vi "re_LuaVIEW Registry Daemon.vi"   [LabVIEW 2012]
doc: "This daemon opens references to public function VIs and manages the public registry. By running in the background it prevents LabVIEW from prematurely closing those references, which happens when the top-level context in which the reference was opened terminates. This daemon is messaged via the \"Daemon Exchange\" object.\n\nThis VI is reentrant so that it can be prepared for a reentrant run which allows it to be run even though it is included into the hierarchy via a static VI reference."
uses:
  typedefs/t_LuaVIEW Registry Daemon States.ctl
  typedefs/t_LuaVIEW Daemon Exchange Methods.ctl
  typedefs/t_LuaVIEW CIN Spinlocked Actions.ctl
  typedefs/t_LuaVIEW Reference.ctl
types:
  T1 = typedef "t_LuaVIEW Daemon Exchange Methods.ctl" = enum16{"inert", "send path", "send cleanup", "get sent", "reply", "get reply", "unset launched"}
  T2 = typedef "t_LuaVIEW Registry Daemon States.ctl" = enum16{"empty queue", "handle message", "exit LabVIEW", "initialize", "cleanup tasks", "cleanup", "stop"}
  T3 = typedef "t_LuaVIEW CIN Spinlocked Actions.ctl" = enum16{"totals", "taskcount", "open", "registerpublic", "registerexport", "revokeexports", "unregnextpublic", "usepublic", "pollexport", "close", "startyieldtest", "endyieldtest", "pollprintbuffer"}
  T4 = typedef "t_LuaVIEW Reference.ctl" = refnum<k1>
  T5 = typedef "et_LuaVIEW CIN Results.ctl" = enum16{"OK", "error", "main", "call", "clonecall", "modulecall", "exportcall", "index", "yield"}
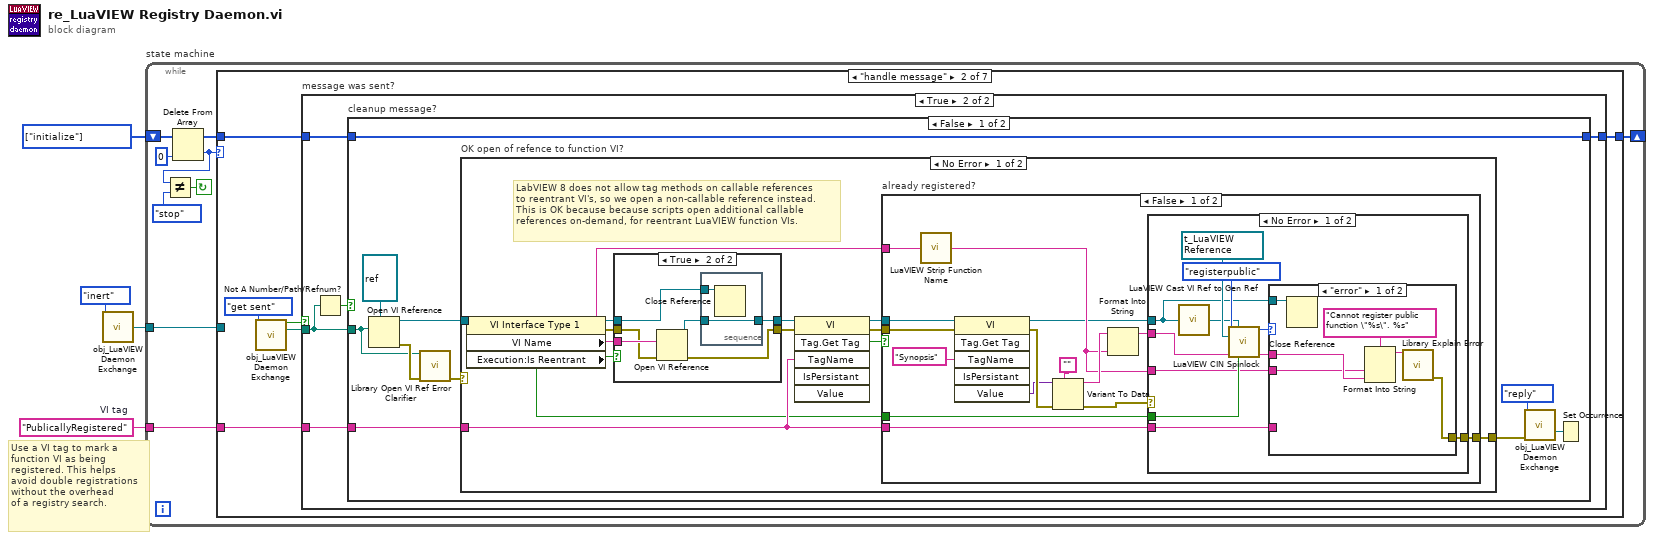
[diagram p0: block diagram]
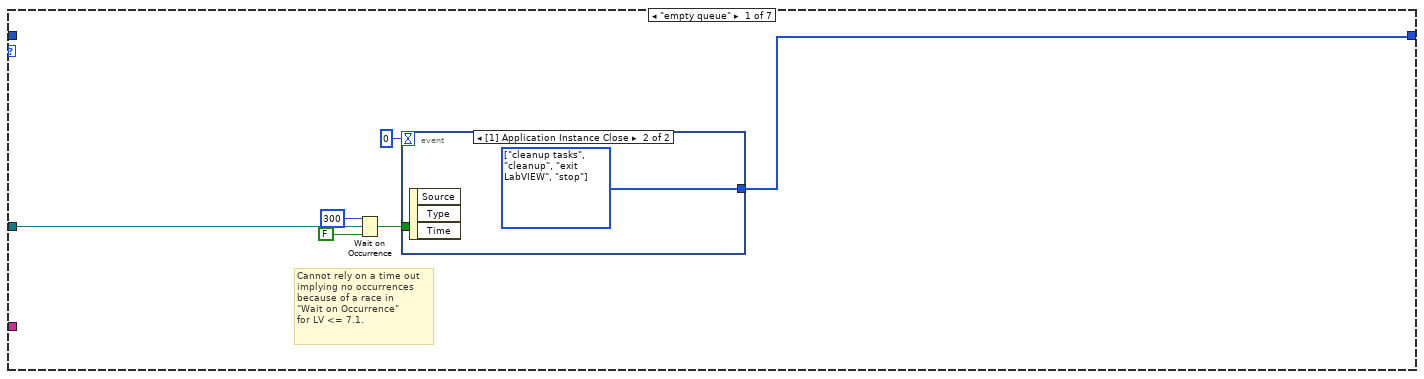
[diagram p2: hidden frame]
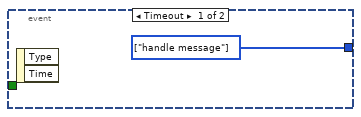
[diagram p3: hidden frame]
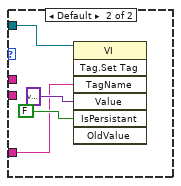
[diagram p6: hidden frame]
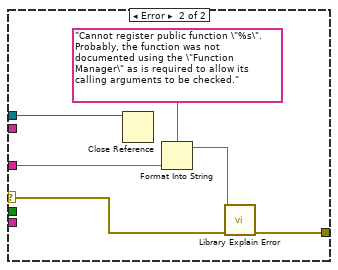
[diagram p7: hidden frame]
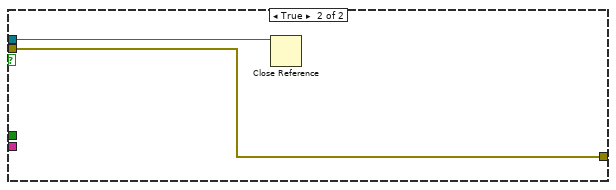
[diagram p8: hidden frame]
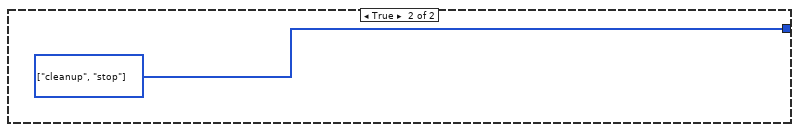
[diagram p10: hidden frame]
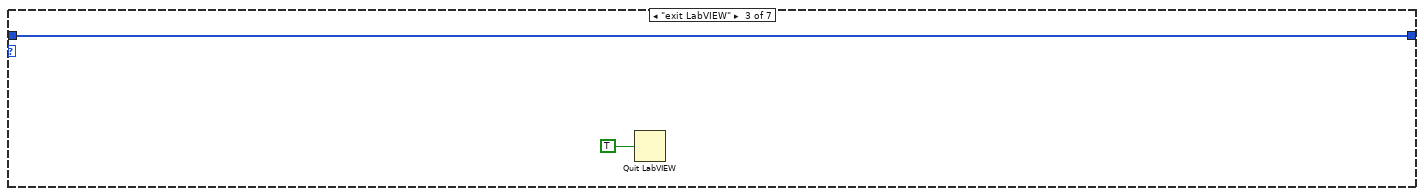
[diagram p11: hidden frame]
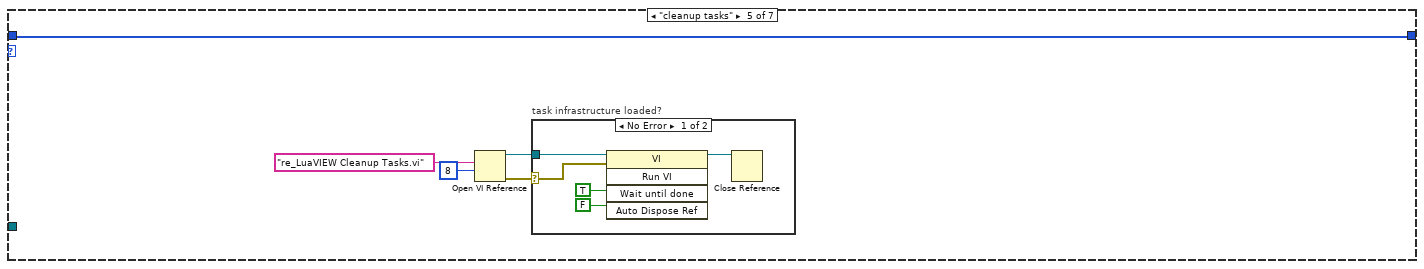
[diagram p13: hidden frame]
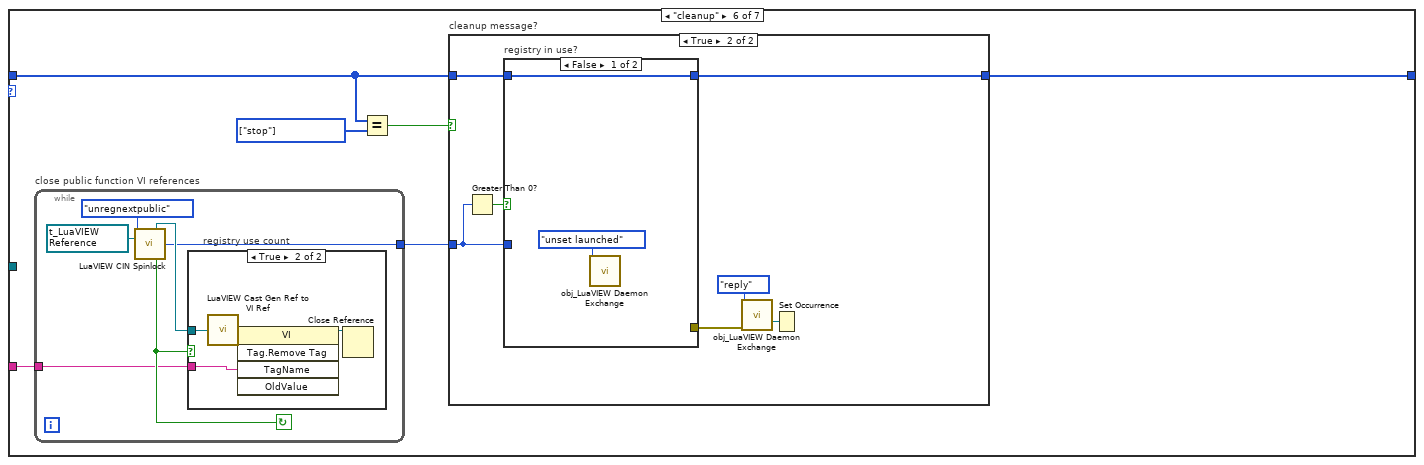
[diagram p15: hidden frame]
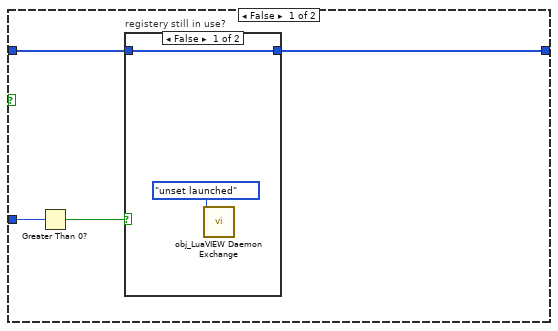
[diagram p16: hidden frame]
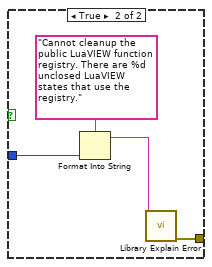
[diagram p18: hidden frame]
diagram:
  w1 = "PublicallyRegistered"  # VI tag
  w4 = T2[] [enum."initialize"] items=["empty queue", "handle message", "exit LabVIEW", "initialize", "cleanup tasks", "cleanup", "stop"] ("Array Constant")
  # "Use a VI tag to mark a\nfunction VI as being\nregistered. This helps\navoid double registrations\nwithout the overhead\nof a registry search."
  n1 = call "obj_LuaVIEW Daemon Exchange.vi"("method"=t_LuaVIEW_Daemon_Exchange_Methods."inert") -> ("send occurrence"=w2:refnum<k4>)  [unwired: 10 in, 4 out]
  n2 = while "state machine" {
    shift-left: w4 -> [w10]
    shift-right: [w13] -> _
    tunnel: w2 -> [w6]
    tunnel: w1 -> [w5]
    stop <- w12 continue-if-true
    n3 = Delete From Array(array=w10, index=0) -> (deleted portion=w8:T2, array with subset deleted=w9:T2[])  [unwired: 1 in]
    n4 = Not Equal?(x=w8, y=t_LuaVIEW_Registry_Daemon_States."stop" ("states")) -> (x != y?=w12:bool)
    n5 = case "Case" shown="\"handle message\"" w8 {
      tunnel: [w16 w23 w113 w114 w119 w130 w160] -> w13
      tunnel: w9 -> [_ w24 w113 w114 w119 w128 w160]
      tunnel: w6 -> [w17 _ _ _ _ _ _]
      tunnel: w5 -> [_ w22 _ _ _ w129 _]
      frame "empty queue" {
        # "Cannot rely on a time out\nimplying no occurrences\nbecause of a race in\n\"Wait on Occurrence\"\nfor LV <= 7.1."
        n6 = Wait on Occurrence(1:FALSE ("ignore previous (T)"), 2:w17, 3:300 ("ms timeout (-1)")) -> (0:w14:bool)
        n7 = event shown="[1] Application Instance Close" {
          selector: _ -> [_ _]
          dyn-events: _ -> [_ _]
          timeout: 0 -> [_ _]
          tunnel: [w20 w21] -> w16
          tunnel: w14 -> [_ _]
          event Timeout {
            w20 = T2[] [enum."handle message"] items=["empty queue", "handle message", "exit LabVIEW", "initialize", "cleanup tasks", "cleanup", "stop"] ("Array Constant")
            n8 = event-data() -> ()  [unwired: 1 in, 2 out]
          }
          event Application Instance Close {
            w21 = T2[] [enum."cleanup tasks", enum."cleanup", enum."exit LabVIEW", enum."stop"] items=["empty queue", "handle message", "exit LabVIEW", "initialize", "cleanup tasks", "cleanup", "stop"] ("Array Constant")
            n9 = event-data() -> ()  [unwired: 1 in, 3 out]
          }
        }
      }
      frame "handle message" {
        n10 = call "obj_LuaVIEW Daemon Exchange.vi"("method"=t_LuaVIEW_Daemon_Exchange_Methods."get sent") -> ("available?"=w25:bool, "path out"=w26:path)  [unwired: 10 in, 3 out]
        n11 = case "message was sent?" shown="True" w25 {
          tunnel: w26 -> [_ w31]
          tunnel: w24 -> [w28 w33]
          tunnel: [w28 w32] -> w23
          tunnel: w22 -> [_ w29]
          frame False {
          }
          frame True {
            n12 = Not A Number/Path/Refnum?(number/path/refnum=w31) -> (NaN/Path/Refnum?=w30:bool)
            n13 = case "cleanup message?" shown="False" w30 {
              tunnel: w31 -> [w42 _]
              tunnel: w33 -> [w41 _]
              tunnel: [w41 w111] -> w32
              tunnel: w29 -> [w38 _]
              frame False {
                n14 = Open VI Reference(type specifier VI Refnum (for type only)=refnum<vi> refnum ("function pane"), vi path=w42) -> (vi reference=w39:refnum<vi>, error out=w43:errorcluster)  [unwired: 4 in]
                n15 = call "Library Open VI Ref Error Clarifier.vi"("VI path"=w42, "called VI error (no error)"=w43) -> ("error out"=w40:errorcluster)  [unwired: 13 in]
                n16 = case "OK open of refence to function VI?" shown="No Error" w40 {
                  selector: w40 -> [_ w110]
                  tunnel: [w55 w110] -> w35
                  tunnel: w39 -> [w50 _]
                  tunnel: w38 -> [w52 _]
                  frame No Error {
                    # "LabVIEW 8 does not allow tag methods on callable references\nto reentrant VI's, so we open a non-callable reference instead.\nThis is OK because because scripts open additional callable\nreferences on-demand, for reentrant LuaVIEW function VIs."
                    n17 = property class="VI Interface Type 1"(reference=w50) -> (reference out=w44:refnum<vi>, error out=w47:errorcluster, "VI Name"=w48:string, "Execution:Is Reentrant"=w49:bool)  [unwired: 1 in]
                    n18 = case shown="True" w49 {
                      tunnel: w48 -> [_ w63]
                      tunnel: w47 -> [w56 w62]
                      tunnel: [w56 w61] -> w46
                      tunnel: [w57 w60] -> w45
                      tunnel: w44 -> [w57 w58]
                      frame False {
                      }
                      frame True {
                        n19 = Open VI Reference(vi path=w63, error in (no error)=w62) -> (vi reference=w59:refnum<vi>, error out=w61:errorcluster)  [unwired: 4 in]
                        n20 = stacked-sequence {
                          tunnel: [w65] -> w60
                          tunnel: w59 -> [w65]
                          tunnel: w58 -> [w64]
                          frame #0 {
                            n21 = Close Reference(reference=w64) -> ()  [unwired: 1 in, 1 out]
                          }
                        }
                      }
                    }
                    n22 = invoke class="VI" method="Tag.Get Tag"(reference=w45, error in=w46, "TagName"=w52) -> (reference out=w51:refnum<vi>, error out=w53:errorcluster, "GetTag"=w54:bool)  [unwired: 3 in, 3 out]
                    n23 = case "already registered?" shown="False" w54 {
                      tunnel: [w79 w108] -> w55
                      tunnel: w51 -> [w67 w109]
                      tunnel: w53 -> [w66 w108]
                      tunnel: w52 -> [w80 _]
                      tunnel: w49 -> [w69 _]
                      tunnel: w48 -> [w68 _]
                      frame False {
                        n24 = call "LuaVIEW Strip Function Name.vi"("function VI name"=w68) -> ("Lua function name"=w72:string)  [unwired: 14 in]
                        n25 = invoke class="VI" method="Tag.Get Tag"(reference=w67, error in=w66, "TagName"="Synopsis") -> (reference out=w71:refnum<vi>, error out=w78:errorcluster, "Value"=w74:variant)  [unwired: 3 in, 3 out]
                        n26 = Variant To Data(error in=w78, type="", Variant=w74) -> (data=w75:string, error out=w70:errorcluster)
                        n27 = Format Into String(format string=w75, w72) -> (resulting string=w73:string)  [unwired: 2 in, 1 out]
                        n28 = case shown="No Error" w70 {
                          selector: w70 -> [_ w103]
                          tunnel: [w90 w102] -> w79
                          tunnel: w71 -> [w84 w107]
                          tunnel: w69 -> [w87 _]
                          tunnel: w80 -> [w85 _]
                          tunnel: w72 -> [w82 w105]
                          tunnel: w73 -> [w81 _]
                          frame No Error {
                            w86 = T4 refnum items=["LuaVIEW"] ("LuaVIEW reference in")
                            n29 = call "LuaVIEW Cast VI Ref to Gen Ref.vi"("refnum in"=w84) -> ("refnum out"=w83:refnum<vi>)  [unwired: 14 in]
                            n30 = call "LuaVIEW CIN Spinlock.vi"("action"=t_LuaVIEW_CIN_Spinlocked_Actions."registerpublic", "refnum in"=w83, "LuaVIEW reference in"=w86, "string in"=w81, "boolean in"=w87) -> ("result"=w91:T5, "string out"=w89:string)  [unwired: 4 in, 5 out]
                            n31 = case shown="\"error\"" w91 {
                              tunnel: [w94 _] -> w90
                              tunnel: w89 -> [w96 _]
                              tunnel: w82 -> [w93 _]
                              tunnel: w84 -> [w92 w99]
                              tunnel: w85 -> [_ w98]
                              frame "error" {
                                n32 = Close Reference(reference=w92) -> ()  [unwired: 1 in, 1 out]
                                n33 = Format Into String(format string="Cannot register public function \"%s\". %s", w93, w96) -> (resulting string=w95:string)  [unwired: 2 in, 1 out]
                                n34 = call "Library Explain Error.vi"("explanation prefix (none)"=w95) -> ("explained error"=w94:errorcluster)  [unwired: 14 in]
                              }
                              frame Default {
                                n35 = invoke class="VI" method="Tag.Set Tag"(reference=w99, "TagName"=w98, "Value"=variant, "IsPersistant"=FALSE) -> ()  [unwired: 3 in, 7 out]
                              }
                            }
                          }
                          frame Error {
                            n36 = Close Reference(reference=w107) -> ()  [unwired: 1 in, 1 out]
                            n37 = Format Into String(format string="Cannot register public function \"%s\". Probably, the function was not  documented using the \"Function Manager\" as is required to allow its calling arguments to be checked.", w105) -> (resulting string=w104:string)  [unwired: 2 in, 1 out]
                            n38 = call "Library Explain Error.vi"("explanation prefix (none)"=w104, "error in (no error)"=w103) -> ("explained error"=w102:errorcluster)  [unwired: 13 in]
                          }
                        }
                      }
                      frame True {
                        n39 = Close Reference(reference=w109) -> ()  [unwired: 1 in, 1 out]
                      }
                    }
                  }
                  frame Error {
                  }
                }
                n40 = call "obj_LuaVIEW Daemon Exchange.vi"("method"=t_LuaVIEW_Daemon_Exchange_Methods."reply", "error reply in"=w35) -> ("reply occurrence"=w37:refnum<k4>)  [unwired: 9 in, 4 out]
                n41 = Set Occurrence(w37) -> ()
              }
              frame True {
                w111 = T2[] [enum."cleanup", enum."stop"] items=["empty queue", "handle message", "exit LabVIEW", "initialize", "cleanup tasks", "cleanup", "stop"] ("Array Constant")
              }
            }
          }
        }
      }
      frame "exit LabVIEW" {
        n42 = Quit LabVIEW(quit? (T)=TRUE) -> ()
      }
      frame "initialize" {
      }
      frame "cleanup tasks" {
        n43 = Open VI Reference(vi path="re_LuaVIEW Cleanup Tasks.vi", options=8) -> (vi reference=w117:refnum<vi>, error out=w115:errorcluster)  [unwired: 4 in]
        n44 = case "task infrastructure loaded?" shown="No Error" w115 {
          selector: w115 -> [w120 _]
          tunnel: w117 -> [w124 _]
          frame No Error {
            n45 = invoke class="VI" method="Run VI"(reference=w124, error in=w120, "Wait until done"=TRUE, "Auto Dispose Ref"=FALSE) -> (reference out=w121:refnum<vi>)  [unwired: 1 in, 4 out]
            n46 = Close Reference(reference=w121) -> ()  [unwired: 1 in, 1 out]
          }
          frame Error {
          }
        }
      }
      frame "cleanup" {
        w127 = T2[] [enum."stop"] items=["empty queue", "handle message", "exit LabVIEW", "initialize", "cleanup tasks", "cleanup", "stop"] ("Array Constant")
        n47 = while "close public function VI references" {
          tunnel: [w152] -> w125
          tunnel: w129 -> [w151]
          stop <- w155 continue-if-true
          w153 = T4 refnum items=["LuaVIEW"] ("LuaVIEW reference in")
          # "registry use count"
          n48 = call "LuaVIEW CIN Spinlock.vi"("action"=t_LuaVIEW_CIN_Spinlocked_Actions."unregnextpublic", "LuaVIEW reference in"=w153) -> ("refnum out"=w154:refnum<vi>, "index out"=w152:i32, "boolean out"=w155:bool)  [unwired: 7 in, 4 out]
          n49 = case shown="True" w155 {
            tunnel: w154 -> [_ w159]
            tunnel: w151 -> [_ w157]
            frame False {
            }
            frame True {
              n50 = call "LuaVIEW Cast Gen Ref to VI Ref.vi"("refnum in"=w159) -> ("refnum out"=w156:refnum<vi>)  [unwired: 14 in]
              n51 = invoke class="VI" method="Tag.Remove Tag"(reference=w156, "TagName"=w157) -> (reference out=w158:refnum<vi>)  [unwired: 3 in, 4 out]
              n52 = Close Reference(reference=w158) -> ()  [unwired: 1 in, 1 out]
            }
          }
        }
        n53 = Equal?(x=w128, y=w127) -> (x = y?=w126:bool)
        n54 = case "cleanup message?" shown="True" w126 {
          tunnel: [w131 w137] -> w130
          tunnel: w128 -> [w132 w138]
          tunnel: w125 -> [w134 w139]
          frame False {
            n55 = Greater Than 0?(x=w134) -> (x > 0?=w133:bool)
            n56 = case "registery still in use?" shown="False" w133 {
              tunnel: w132 -> [w135 _]
              tunnel: [w135 _] -> w131
              frame False {
                n57 = call "obj_LuaVIEW Daemon Exchange.vi"("method"=t_LuaVIEW_Daemon_Exchange_Methods."unset launched") -> ()  [unwired: 10 in, 5 out]
              }
              frame True {
              }
            }
          }
          frame True {
            n58 = Greater Than 0?(x=w139) -> (x > 0?=w140:bool)
            n59 = case "registry in use?" shown="False" w140 {
              tunnel: [_ w149] -> w141
              tunnel: w139 -> [_ w148]
              tunnel: w138 -> [w145 _]
              tunnel: [w145 _] -> w137
              frame False {
                n60 = call "obj_LuaVIEW Daemon Exchange.vi"("method"=t_LuaVIEW_Daemon_Exchange_Methods."unset launched") -> ()  [unwired: 10 in, 5 out]
              }
              frame True {
                n61 = Format Into String(format string="Cannot cleanup the public LuaVIEW function registry. There are %d unclosed LuaVIEW states that use the registry." ("explanation"), w148) -> (resulting string=w146:string)  [unwired: 2 in, 1 out]
                n62 = call "Library Explain Error.vi"("explanation prefix (none)"=w146) -> ("explained error"=w149:errorcluster)  [unwired: 14 in]
              }
            }
            n63 = call "obj_LuaVIEW Daemon Exchange.vi"("method"=t_LuaVIEW_Daemon_Exchange_Methods."reply", "error reply in"=w141) -> ("reply occurrence"=w142:refnum<k4>)  [unwired: 9 in, 4 out]
            n64 = Set Occurrence(w142) -> ()
          }
        }
      }
      frame "stop" {
      }
    }
  }
